vi "PeformSelfTest.vi"(8 "Fehler (Eingang, kein Fehler)":errorcluster caption="Error_In", 11 "OXYGEN Ref In":refnum<visa-resource-name>) -> (0 "Fehler (Ausgang)":errorcluster caption="Error_Out", 1 "communication_data":T1, 2 "Register State":u32, 3 "OXYGEN Ref Out":refnum<visa-resource-name>)   [LabVIEW 2018, in "OXYGEN.lvlib"]
doc: "Performs a self-test and queries the result."
uses:
  OXYGEN.lvlib
  TypeDefs/Cluster_RawCommData.ctl
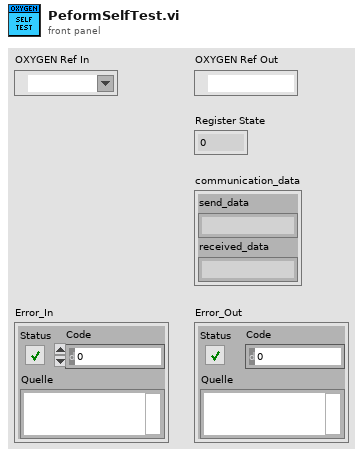
[diagram p1: front panel]
types:
  T1 = typedef "OXYGEN.lvlib/Cluster_RawCommData.ctl" = cluster{"send_data":string, "received_data":string}
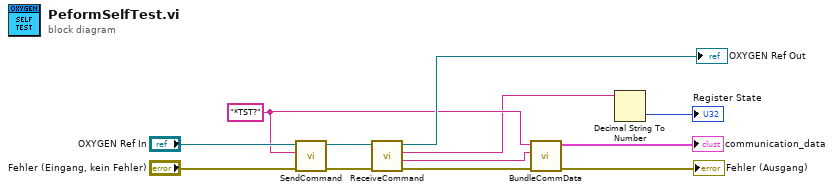
[diagram p0: block diagram]
diagram:
  w7 = "*TST?" ("Schreibpuffer")
  n1 = call "SendCommand.vi"("error in (no error)"="Fehler (Eingang, kein Fehler)", "String to Send"=w7, "OXY_SCPI Reseource In"="OXYGEN Ref In") -> ("error out"=w9:errorcluster, "OXY_SCPI Reseource Out"=w8:refnum<visa-resource-name>)  [unwired: 7 in]
  n2 = call "ReceiveCommand.vi"("error in (no error)"=w9, "OXY_SCPI Reseource In"=w8) -> ("error out"=w4:errorcluster, "received Data with Header"=w1:string, "received Data"=w6:string, "OXY_SCPI Reseource Out"=→"OXYGEN Ref Out":refnum<visa-resource-name>)  [unwired: 6 in]
  n3 = call "BundleCommData.vi"("error in (no error)"=w4, "received_data"=w1, "send_data"=w7) -> ("error out"=→"Fehler (Ausgang)":errorcluster, "communication_data"=→"communication_data":T1)  [unwired: 7 in]
  n4 = Decimal String To Number(string=w6) -> (number=→"Register State":i32)  [unwired: 2 in, 1 out]
